vi "Glimpse Generate Test Sequence.vi"() -> ()   [LabVIEW 2011]
uses:
  Sequence files handle.ctt
  Header2 file data.ctl
  Seq file v 1/Offset table.ctl
  Seq file v 1/Offset.ctl
  Seq file v 1/file number.ctl
  GLIMPSE Globals.vi
  <vilib>/vision/NI_Vision_Development_Module.lvlib
panel:
  in  "Number of frames to make":i32=20
  in  "Go? (F)":bool
  in  "New":bool
  in  "Over-write":bool=TRUE
  in  "Over-write exisitng:":path=path "d:/1.glimpse"
  in  "Digitize to new directory":path=path "d:/1.glimpse"
  in  "stop":bool
  out "Frames created":u32(slide) scale=0.0..20.0
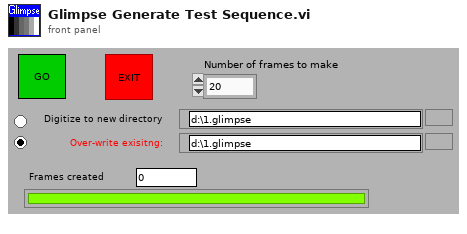
[diagram p1: front panel]
types:
  T1 = enum32{"8 bits", "16 bits", "Float", "Complex", "RGB Chunky", "Compressed"}
  T2 = typedef "Sequence files handle.ctt" = cluster{"Sequence files directory path":path, "Sequence files refnum array":refnum<file>[]}
  T3 = typedef "Offset table.ctl" = cluster{"offset":T4, "file number":T5}[]
  T4 = typedef "Offset.ctl" = i32
  T5 = typedef "file number.ctl" = u8
  T6 = enum32{"Frame", "Paint", "Invert Frame", "Invert Paint"}
  T7 = cluster{"desired font(Application)":enum16{"User-specified Font", "Application Font", "System Font", "Dialog Font"}, "[user-specified font]":cluster{"Font Name:":string, "Size":i16, "Strikeout?":bool, "Italic?":bool, "Underline?":bool, "Outline?":bool, "Shadow?":bool, "Bold?":bool}, "Alignment":i32}
  T8 = typedef "Header2 file data.ctl" = cluster{"Camera":string, "Microscope":string, "Microscope software version":string, "Laser names":string[], "Filter names":string[], "Lasers array":u16[][], "Filter array":u16[], "Flow rate array":dbl[], "Temperature array":dbl[], "Field array":u16[], "Is header2 info present?":bool, "Description Info":string, "Stage xyz array":dbl[][]}
  T9 = typedef "IMAQ Image.ctl" = refnum<image>
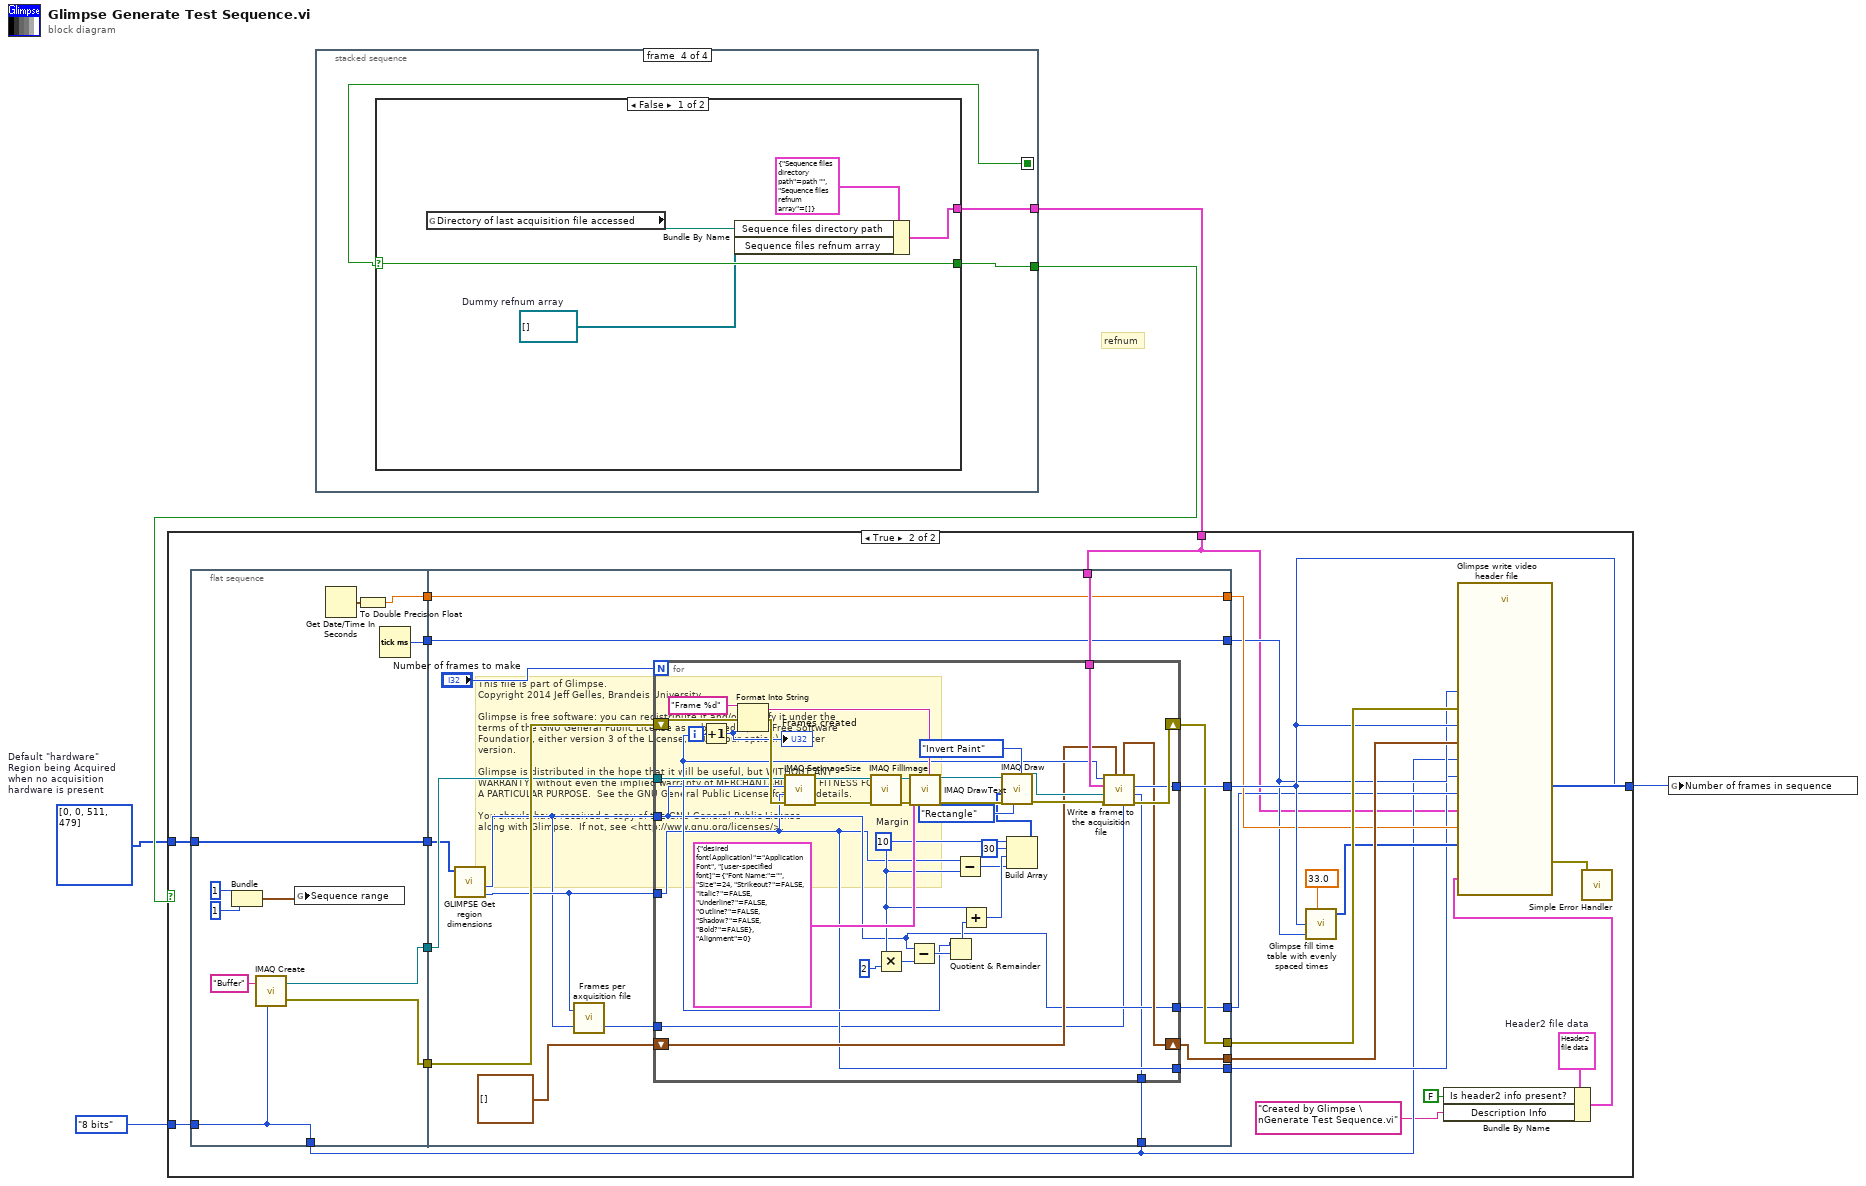
[diagram p0: block diagram]
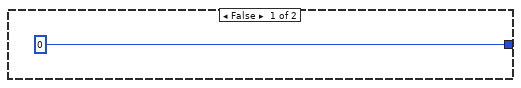
[diagram p2: hidden frame]
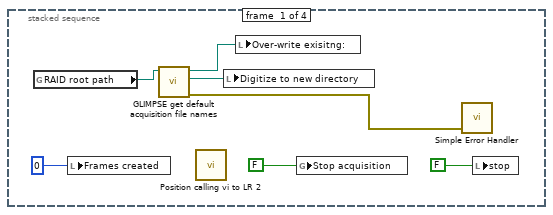
[diagram p3: hidden frame]
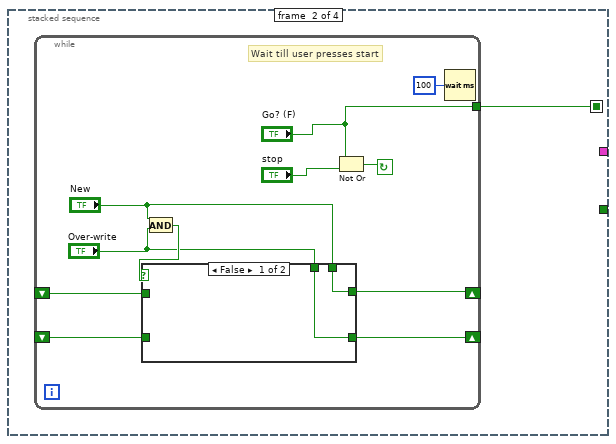
[diagram p4: hidden frame]
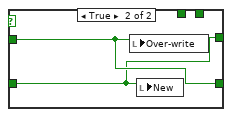
[diagram p5: hidden frame]
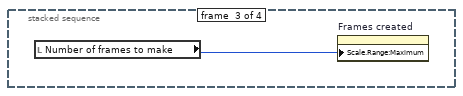
[diagram p6: hidden frame]
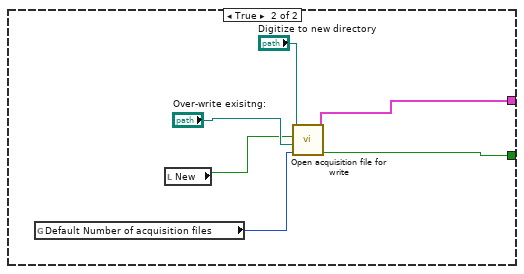
[diagram p7: hidden frame]
diagram:
  w2 = i32[] [0, 0, 511, 479]  # Default "hardware" Region being Acquired when no acquisition hardware is present
  # "This file is part of Glimpse. \nCopyright 2014 Jeff Gelles, Brandeis University.    \n\nGlimpse is free software: you can redistribute it and/or modify it under the \nterms of the GNU General Public License as published by the Free Software \nFoundation, either version 3 of the License, or (at your option) any later \nversion.\n\nGlimpse is distributed in the hope that it will be useful, but WITHOUT ANY \nWARRANTY; without even the implied warranty of MERCHANTABILITY or FITNESS FOR \nA PARTICULAR PURPOSE.  See the GNU General Public License for more details.\n\nYou should have received a copy of the GNU General Public License\nalong with Glimpse.  If not, see <http://www.gnu.org/licenses/>."
  # "refnum"
  n1 = stacked-sequence {
    seq-local: [_ w13 _ _] -> [_ _ _ w32]
    tunnel: [_ _ _ w31] -> w5
    tunnel: [_ _ _ w30] -> w3
    frame #0 {
      n2 = global read "GLIMPSE Globals.vi" "RAID root path"() -> (w10:path)
      n3 = local write "Frames created"(u32 0 ("Frames Acquired")) -> ()
      n4 = call "GLIMPSE get default acquisition file names.vi"("RAID root path"=w10) -> ("error out"=w9:errorcluster, "next directory path"=w8:path, "last directory path"=w7:path)  [unwired: 1 in, 5 out]
      n5 = call "Position calling vi to LR 2.vi"() -> ()  [unwired: 2 in, 4 out]
      n6 = local write "Digitize to new directory"(w8) -> ()
      n7 = local write "Over-write exisitng:"(w7) -> ()
      n8 = global write "GLIMPSE Globals.vi" "Stop acquisition"(FALSE ("Stop acquisition")) -> ()
      n9 = call <vilib>:"Simple Error Handler.vi"("error in (no error)"=w9) -> ()  [unwired: 1 in, 8 out]
      n10 = local write "stop"(FALSE ("stop")) -> ()
    }
    frame #1 {
      n11 = while {
        tunnel: ["Go? (F)"] -> w13
        shift-right: [w20] -> _
        shift-left: _ -> [w17]
        shift-right: [w18] -> _
        shift-left: _ -> [w16]
        stop <- w24 continue-if-true
        # "Wait till user presses start"
        n12 = And(x="New", y="Over-write") -> (x .and. y?=w22:bool)
        n13 = case shown="False" w22 {
          tunnel: [w26 w27] -> w20
          tunnel: "New" -> [w26 _]
          tunnel: "Over-write" -> [w25 _]
          tunnel: [w25 w28] -> w18
          tunnel: w17 -> [_ w28]
          tunnel: w16 -> [_ w27]
          frame False {
          }
          frame True {
            n14 = local write "Over-write"(w28) -> ()
            n15 = local write "New"(w27) -> ()
          }
        }
        n16 = Not Or(1:"stop", 2:"Go? (F)") -> (0:w24:bool)
        n17 = Wait (ms)(milliseconds to wait=u32 100) -> ()  [unwired: 1 out]
      }
    }
    frame #2 {
      n18 = local read "Number of frames to make"() -> (w29:i32)
      n19 = property on="Frames created" class="Slide (strict)"("Scale.Range:Maximum"=w29) -> ()  [unwired: 2 in, 2 out]
    }
    frame #3 {
      n20 = case shown="False" w32 {
        selector: w32 -> [w37 _]
        tunnel: [w37 w43] -> w31
        tunnel: [w34 w38] -> w30
        frame False {
          w35 = refnum<file>[] []  # Dummy refnum array
          n21 = global read "GLIMPSE Globals.vi" "Directory of last acquisition file accessed"() -> (w36:path)
          n22 = Bundle By Name(cluster=T2 {"Sequence files directory path"=path "", "Sequence files refnum array"=[]} ("Sequence files handle"), "Sequence files directory path"=w36, "Sequence files refnum array"=w35) -> (w34:T2)
        }
        frame True {
          n23 = global read "GLIMPSE Globals.vi" "Default Number of acquisition files"() -> (w39:i32)
          n24 = local read "New"() -> (w40:bool)
          n25 = call "Open acquisition file for write.vi"("Number of acquisition files"=w39, "Existing directory to over-write"="Over-write exisitng:", "Use new?"=w40, "New directory to create"="Digitize to new directory") -> ("OK?"=w43:bool, "Sequence files handle"=w38:T2)  [unwired: 5 out]
        }
      }
    }
  }
  n26 = case shown="True" w5 {
    tunnel: [u32 0 ("Last frame number written out") w62] -> w4
    tunnel: w3 -> [_ w49]
    tunnel: w2 -> [_ w64]
    tunnel: T1."8 bits" ("Image Type") -> [_ w55]
    frame False {
    }
    frame True {
      w48 = T8 {"Camera"="", "Microscope"="", "Microscope software version"="", "Laser names"=[], "Filter names"=[], "Lasers array"=[], "Filter array"=[], "Flow rate array"=[], "Temperature array"=[], "Field array"=[], "Is header2 info present?"=FALSE, "Description Info"="", "Stage xyz array"=[]}  # Header2 file data
      n27 = flat-sequence {
        tunnel: w64 -> [w69]
        tunnel: [w69] -> w60
        tunnel: [w78] -> w59
        tunnel: [w73] -> w58
        tunnel: [w72] -> w57
        tunnel: [w70] -> w56
        tunnel: w55 -> [w68]
        tunnel: [w68] -> w50
        tunnel: [w93] -> w62
        tunnel: [w91] -> w67
        tunnel: [w90] -> w65
        tunnel: w60 -> [w88]
        tunnel: w59 -> [w86]
        tunnel: w58 -> [w94]
        tunnel: w57 -> [w95]
        tunnel: w56 -> [w85]
        tunnel: w49 -> [w87]
        tunnel: [w86] -> w53
        tunnel: [w85] -> w54
        tunnel: [w84] -> w52
        tunnel: [w83] -> w51
        tunnel: w50 -> [w82]
        frame #0 {
          n28 = Bundle(i16 1, i16 1) -> (w77:cluster{i16, i16})  [unwired: 1 out]
          n29 = call "IMAQ Create"("Image Name"="Buffer", "Image Type"=w68) -> ("New Image"=w73:T9, "error out"=w72:errorcluster)  [unwired: 2 in, 1 out]
          n30 = global write "GLIMPSE Globals.vi" "Sequence range"(w77) -> ()
          n31 = Get Date/Time In Seconds() -> (seconds since 1Jan1904=w71:timestamp)
          n32 = To Double Precision Float(number=w71) -> (double precision float=w70:dbl)
          n33 = Tick Count (ms)() -> (millisecond timer value=w78:u32)
        }
        frame #1 {
          n34 = call "GLIMPSE Get region dimensions.vi"("x1y1x2y2"=w88) -> ("y size"=w81:u16, "x size"=w80:u16)  [unwired: 9 out]
          n35 = call "Frames per axquisition file.vi"("Output frame width"=w80, "Output frame height"=w81) -> ("Frames per acquisition file"=w79:i32)  [unwired: 1 out]
          n36 = for {
            N: "Number of frames to make" -> [_]
            shift-right: [w106] -> w90
            shift-left: w95 -> [w130]
            tunnel: w80 -> [w99]
            tunnel: w81 -> [w98]
            tunnel: w94 -> [w108]
            tunnel: w87 -> [w104]
            tunnel: [w103] -> w93
            shift-right: [w100] -> w91
            shift-left: T3 [] ("Offset table in") -> [w101]
            tunnel: [w99] -> w84
            tunnel: [w98] -> w83
            tunnel: w82 -> [w97]
            tunnel: w79 -> [w96]
            i -> [w102]
            w111 = 10  # Margin
            n37 = Increment(x=w102) -> (x+1=w109:i32)
            "Frames created" <- w109
            n38 = Format Into String(format string="Frame %d", error in=w130, w109) -> (resulting string=w129:string, error out=w124:errorcluster)  [unwired: 1 in]
            n39 = call "IMAQ SetImageSize"("error in (no error)"=w124, "Y Resolution"=w98, "X Resolution"=w99, "Image"=w108) -> ("error out"=w126:errorcluster, "Image Out"=w125:T9)  [unwired: 1 out]
            n40 = call "IMAQ FillImage"("error in (no error)"=w126, "Image"=w125) -> ("error out"=w128:errorcluster, "Image Out"=w127:T9)  [unwired: 5 in, 3 out]
            n41 = Multiply(x=w111, y=2) -> (x*y=w115:i32)
            n42 = Subtract(x=w99, y=w115) -> (x-y=w114:i32)
            n43 = call "IMAQ DrawText"("String"=w129, "error in (no error)"=w128, "Font, Size & Style"=T7 {"desired font(Application)"=enum."Application Font", "[user-specified font]"={"Font Name:"="", "Size"=24, "Strikeout?"=FALSE, "Italic?"=FALSE, "Underline?"=FALSE, "Outline?"=FALSE, "Shadow?"=FALSE, "Bold?"=FALSE}, "Alignment"=0}, "Image Src"=w127) -> ("error out"=w122:errorcluster, "Image Dst Out"=w121:T9)  [unwired: 3 in, 3 out]
            n44 = Quotient & Remainder(x=w102, y=w114) -> (x-y*floor(x/y)=w113:i32)  [unwired: 1 out]
            n45 = Subtract(x=w98, y=w111) -> (x-y=w110:i32)
            n46 = Add(x=w111, y=w113) -> (x+y=w112:i32)
            n47 = Build Array(w111, 30 ("Margin"), w112, w110) -> (w118:i32[])
            n48 = call "IMAQ Draw"("Draw Mode"=T6."Invert Paint", "Shape to draw"=enum32{"Line", "Rectangle", "Oval"}."Rectangle", "error in (no error)"=w122, "Coordinates"=w118, "Image Src"=w121) -> ("error out"=w107:errorcluster, "Image Dst Out"=w105:T9)  [unwired: 2 in, 3 out]
            n49 = call "Write a frame to the acquisition file.vi"("Pixel depth"=w97, "Frames per acquisition file"=w96, "Offset table in"=w101, "error in"=w107, "Image In"=w105, "Sequence files handle"=w104, "Last frame number written in"=w102) -> ("error out"=w106:errorcluster, "Last frame number written out"=w103:u32, "Offset table out"=w100:T3)  [unwired: 2 out]
          }
        }
      }
      n50 = call "Glimpse fill time table with evenly spaced times.vi"("Element 0 of TTB"=w53, "Number of frames in sequence"=w62, "Milliseconds per frame"=33.0) -> ("TTB Array"=w61:u32[])  [unwired: 2 out]
      n51 = Bundle By Name(cluster=w48, "Is header2 info present?"=FALSE, "Description Info"="Created by Glimpse \nGenerate Test Sequence.vi") -> (w45:T8)
      n52 = call "Glimpse write video header file.vi"("Number of frames"=w62, "Sequence files handle"=w49, "Pixel depth\n(0=8 bit; 1= 16 bit)"=w50, "error in"=w65, "TTB Array"=w61, "Offsets Array"=w67, "Header2 file data"=w45, "Region width"=w52, "Region height"=w51, "Element 0 of TTB"=w53, "time of 1st frame, \nsec since 1/1/04"=w54) -> ("error out"=w66:errorcluster)  [unwired: 8 in]
      n53 = call <vilib>:"Simple Error Handler.vi"("error in (no error)"=w66) -> ()  [unwired: 1 in, 8 out]
    }
  }
  n54 = global write "GLIMPSE Globals.vi" "Number of frames in sequence"(w4) -> ()
